vi "Constructor.vi"(11 "Espresso in":refnum<class "Espresso.lvclass">) -> (3 "Espresso out":refnum<class "Espresso.lvclass">)   [LabVIEW 2011, in "Espresso.lvclass"]
uses:
  Espresso.lvclass
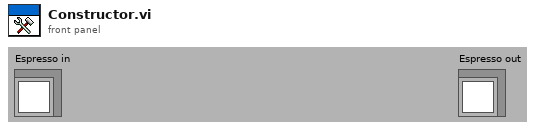
[diagram p1: front panel]
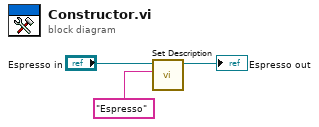
[diagram p0: block diagram]
diagram:
  n1 = call-dynamic "Set Description.vi"("Description"="Espresso", "Beverage in"="Espresso in") -> ("Beverage out"=→"Espresso out":refnum<class "Espresso.lvclass">)  [unwired: 9 in]
